vi "voltage_to_pressure.vi"(11 "Voltage In":dbl[](array[numeric])) -> (1 "Pressure Out":dbl[](array[numeric]), 2 "Coeff Out":dbl[](array[numeric]), 3 "Decade Out":dbl[](array[numeric]))   [LabVIEW 2011]
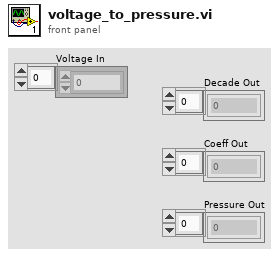
[diagram p1: front panel]
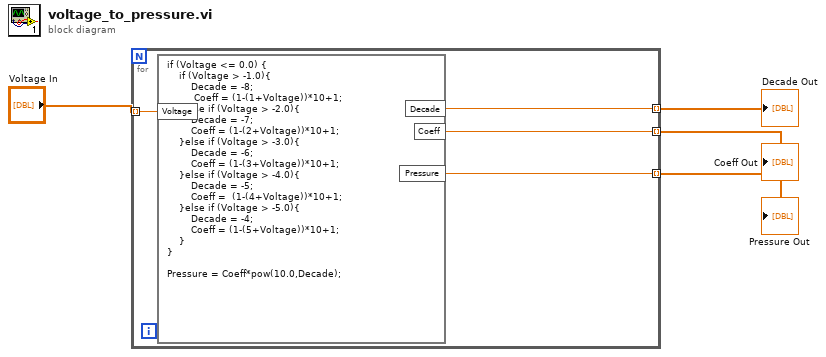
[diagram p0: block diagram]
diagram:
  n1 = for {
    tunnel: [w8] -> w4 mode=indexing
    tunnel: "Voltage In" -> [w7] mode=indexing
    tunnel: [w6] -> w3 mode=indexing
    tunnel: [w5] -> w2 mode=indexing
    n2 = formula code="if (Voltage <= 0.0) {\n    if (Voltage > -1.0){\n        Decade = -8;\n         Coeff = (1-(1+Voltage))*10+1;\n    }else if (Voltage > -2.0){\n        Decade = -7;\n        Coeff = (1-(2+Voltage))*10+1;\n    }else if (Voltage > -3.0){\n        Decade = -6;\n        Coeff = (1-(3+Voltage))*10+1;\n    }else if (Voltage > -4.0){\n        Decade = -5;\n        Coeff =  (1-(4+Voltage))*10+1;\n    }else if (Voltage > -5.0){\n        Decade = -4;\n        Coeff = (1-(5+Voltage))*10+1;\n    }\n}\n\nPressure = Coeff*pow(10.0,Decade);"("Voltage"=w7) -> ("Decade"=w5:dbl, "Coeff"=w6:dbl, "Pressure"=w8:dbl)
  }
  "Pressure Out" <- w4
  "Coeff Out" <- w3
  "Decade Out" <- w2
